vi "ERD_Data_Frame.vi"(0 "Frame":string) -> (4 "Data":string, 8 "ERD":string)   [LabVIEW 2021]
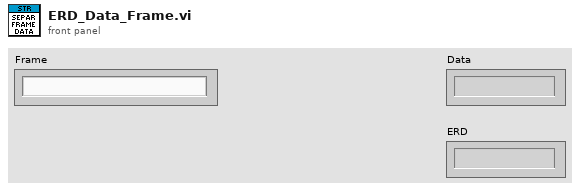
[diagram p1: front panel]
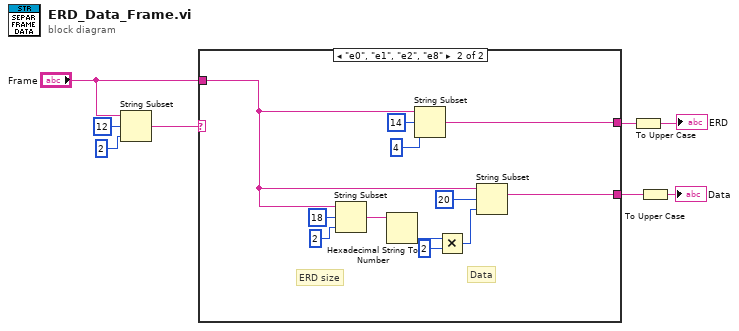
[diagram p0: block diagram]
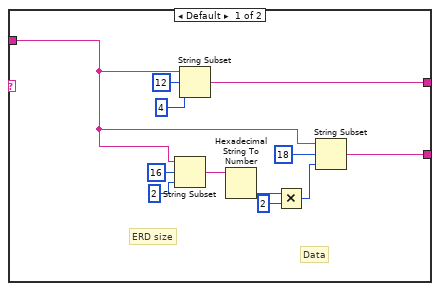
[diagram p2: hidden frame]
diagram:
  n1 = String Subset(string="Frame", offset (0)=12, length (rest)=2 ("length (rest)")) -> (substring=w6:string)
  n2 = case shown="\"e0\", \"e1\", \"e2\", \"e8\"" w6 {
    tunnel: "Frame" -> [w10 w22]
    tunnel: [w18 w30] -> w1
    tunnel: [w9 w21] -> w4
    frame Default {
      # "Data"
      # "ERD size"
      n3 = String Subset(string=w10, offset (0)=16, length (rest)=2 ("length (rest)")) -> (substring=w15:string)
      n4 = String Subset(string=w10, offset (0)=12, length (rest)=4 ("length (rest)")) -> (substring=w18:string)
      n5 = Hexadecimal String To Number(string=w15) -> (number=w16:u32)  [unwired: 2 in, 1 out]
      n6 = Multiply(x=w16, y=u32 2) -> (x*y=w17:u32)
      n7 = String Subset(string=w10, offset (0)=18, length (rest)=w17) -> (substring=w9:string)
    }
    frame "e0", "e1", "e2", "e8" {
      # "Data"
      # "ERD size"
      n8 = String Subset(string=w22, offset (0)=18, length (rest)=2 ("length (rest)")) -> (substring=w27:string)
      n9 = Hexadecimal String To Number(string=w27) -> (number=w28:u32)  [unwired: 2 in, 1 out]
      n10 = String Subset(string=w22, offset (0)=14, length (rest)=4 ("length (rest)")) -> (substring=w30:string)
      n11 = Multiply(x=w28, y=u32 2) -> (x*y=w29:u32)
      n12 = String Subset(string=w22, offset (0)=20, length (rest)=w29) -> (substring=w21:string)
    }
  }
  n13 = To Upper Case(1:w1) -> (0:→"ERD":string)
  n14 = To Upper Case(1:w4) -> (0:→"Data":string)
